vi "Core_Get Notifier.vi"(8 "error in (no error)":errorcluster, 11 "HSMS Class in":refnum<class "HSMS Class.lvclass">) -> (0 "error out":errorcluster, 2 "Notifier Data":T1={"Notifier Type"=enum."Receive Message", "Data"=variant, "Time"=timestamp(0 s since 1904-01-01)}, 3 "HSMS Class out":refnum<class "HSMS Class.lvclass">)   [LabVIEW 2020, in "SECS Communication.lvlib" / "HSMS Class.lvclass"]
uses:
  HSMS Class.lvclass
  Notifier Data.ctl
  Notifier Type.ctl
  HSMS Class.lvclass/HSMS Class.ctl
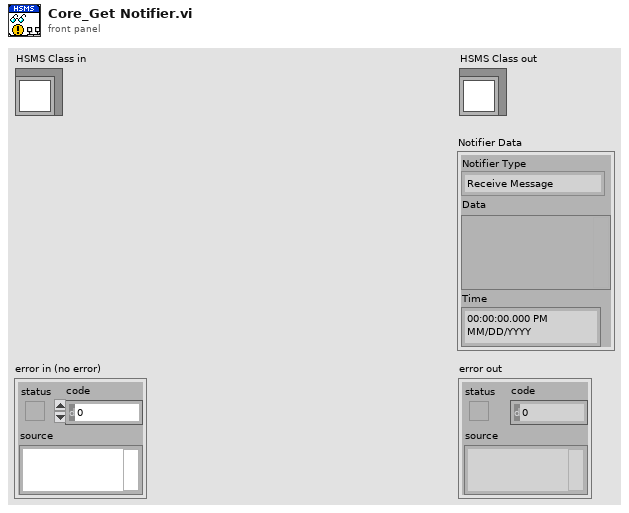
[diagram p1: front panel]
types:
  T1 = typedef "SECS Communication.lvlib/HSMS Class.lvclass/Notifier Data.ctl" = cluster{"Notifier Type":T2, "Data":variant, "Time":timestamp}
  T2 = typedef "SECS Communication.lvlib/HSMS Class.lvclass/Notifier Type.ctl" = enum16{"TCPIP Connect", "TCPIP Disconnect", "Receive Message", "Send Message", "T3 Timeout", "T6 Timeout", "T7 Timeout", "Error", "Stop"}
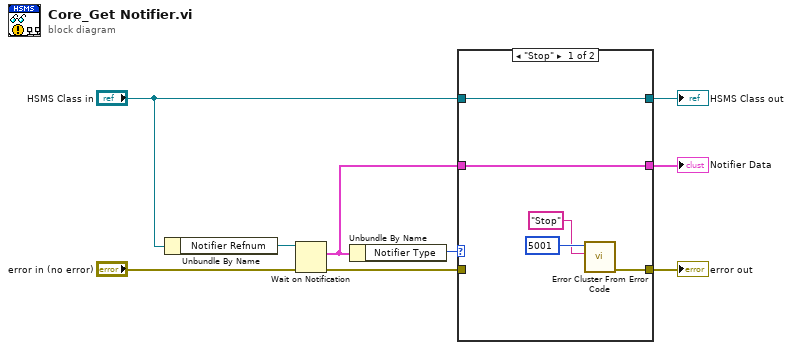
[diagram p0: block diagram]
diagram:
  n1 = Unbundle By Name("HSMS Class in") -> ("Notifier Refnum"=w9:refnum<notifier>)
  n2 = Wait on Notification(notifier=w9, error in (no error)="error in (no error)") -> (notification=w3:T1, error out=w4:errorcluster)  [unwired: 2 in, 2 out]
  n3 = Unbundle By Name(w3) -> ("Notifier Type"=w5:T2)
  n4 = case shown="\"Stop\"" w5 {
    tunnel: "HSMS Class in" -> [w14 w17]
    tunnel: [w14 w17] -> w6
    tunnel: w4 -> [_ w15]
    tunnel: w3 -> [w13 w16]
    tunnel: [w13 w16] -> w2
    tunnel: [w12 w15] -> w1
    frame "Stop" {
      n5 = call <vilib>:"Error Cluster From Error Code.vi"("error message (\"\")"="Stop" ("error message (\"\")"), "error code (0)"=5001) -> ("error out"=w12:errorcluster)  [unwired: 7 in]
    }
    frame Default {
    }
  }
  "error out" <- w1
  "HSMS Class out" <- w6
  "Notifier Data" <- w2
